vi "Intellirupter_tester.vi"() -> ()   [LabVIEW 2016]
uses:
  <vilib>/rvi/interface/nirviCloseFPGA/nirviCloseFPGA.xnode
  <vilib>/rvi/interface/nirviOpenFPGA/nirviOpenFPGA.xnode
  <vilib>/rvi/interface/nirviReadWriteControl/nirviReadWriteControl.xnode
  <vilib>/rvi/interface/Simulation/niFpgaSimulationCallBeginRW.vi
  <vilib>/rvi/errors/niLvFpgaAdjustHostInterfaceError.vi
  FPGA Bitfiles/IntelliRupter_calibrated.lvbitx
  NiFpgaLv.dll
  <vilib>/Utility/error.llb/Error Cluster From Error Code.vi
  <vilib>/FPGAPlugInAG/Dynamic/niLvFpga_Close_Dynamic.vi
  <vilib>/addons/Electrical Power/Protection/Definite Time Delay/subVIs/fpga_Time Delay Cfg.ctl
  <vilib>/addons/Electrical Power/Protection/NI_EP_Protection_FPGA.lvlib
  <vilib>/FPGAPlugInAG/cRIO-9039 (Sync)/niLvFpga_Open_cRIO-9039 (Sync).vi
  <vilib>/rvi/interface/common/dynamic/niFpgaDynamicAddResources.vi
panel:
  out "Protection settings for PV/BESS":T2
  out "dt":sgl
  out "x-y":u32
  in  "Recloser Settings":T3={"Magnitude Minimum"=0.1, "Magnitude difference level"=0.005, "Frequency difference level"=0.1, "Phase difference level"=4.0}
  out "Trip Relay8":bool=TRUE
  out "Trip Relay7":bool=TRUE
  out "Trip Relay6":bool=TRUE
  out "Trip Relay5":bool=TRUE
  out "Trip Relay4":bool=TRUE
  out "Trip Relay3":bool=TRUE
  out "Trip Relay2":bool=TRUE
  out "Trip Relay1":bool=TRUE
  out "MGCC_to_relay":bool[](array[boolean])
  out "Waveform Chart":dbl(graph)=-34.401058197021484
  in  "Count(ticks)":u32=10000
  in  "RMS minimum\nvalues":T4={"VRMS values"=[0.5, 0.5, 0.5], "IRMS values"=[0.1, 0.1, 0.1]}
  out "error out":errorcluster
  out "Relay_toMGCC":bool[](array[boolean])
  in  "Manual trip Relay8":bool
  in  "Reclose Relay8?":bool
  out "R8 Data for\ncommunication":dbl[](array[numeric])=[0.0, 0.0009045934917091171, 0.0009314979378781807, 60.0, 60.0, 28.24567985534668, 1.973525131133958e-08, -4.067070097016323e-08, 0.0, 0.0]
  in  "Manual trip Relay7":bool
  in  "Reclose Relay7?":bool
  out "R7 Data for\ncommunication":dbl[](array[numeric])=[0.0, 0.0007946116254270471, 0.0007993335901335273, 60.0, 60.0, -34.401058197021484, 1.651500881803561e-08, 8.800402599184338e-08, 0.0, 0.0]
  in  "Manual trip Relay6":bool
  in  "Reclose Relay6?":bool
  out "R6 Data for\ncommunication":dbl[](array[numeric])=[0.0, 0.0005957332732847613, 0.0007855918529021252, 60.0, 60.0, 18.105693817138672, 2.5628369915356105e-08, 3.530453627182609e-09, 0.0, 0.0]
  in  "Manual trip Relay5":bool
  in  "Reclose Relay5?":bool
  out "R5 Data for\ncommunication":dbl[](array[numeric])=[0.0, 0.0006951849487988348, 0.0008903021851711478, 60.0, 60.0, -1.4310243129730225, -8.356675233942401e-10, -1.8337251119669163e-09, 0.0, 0.0]
  in  "Manual trip Relay4":bool
  in  "Reclose Relay4?":bool
  out "R4 Data for\ncommunication":dbl[](array[numeric])=[0.0, 0.0007291746865854036, 0.0006235449784023129, 60.0, 60.0, -0.058011382818222046, -5.813950986281207e-08, -7.696689957041477e-08, 0.0, 0.0]
  in  "Manual trip Relay3":bool
  in  "Reclose Relay3?":bool
  out "R3 Data for\ncommunication":dbl[](array[numeric])=[0.0, 0.0007264402728679518, 0.0006124272449413167, 60.0, 60.0, 1.7191237211227417, 2.5547999625248733e-08, -4.286027792555224e-08, 0.0, 0.0]
  in  "Manual trip Relay2":bool
  in  "Reclose Relay2?":bool
  out "R2 Data for\ncommunication":dbl[](array[numeric])=[0.0, 0.0005227375364730379, 0.0005963174374576894, 60.0, 60.0, -1.561047911643982, -2.6251873275059558e-08, 8.429806929664172e-09, 0.0, 0.0]
  out "R1 Data for\ncommunication":dbl[](array[numeric])=[0.0, 0.0006394769755315334, 0.0006284021563432197, 60.0, 60.0, -13.953559875488281, -5.5463867419303074e-08, 7.039235159901093e-08, 0.0, 0.0]
  in  "Relay8":bool
  in  "Relay7":bool
  in  "Relay6":bool
  in  "Relay5":bool
  in  "Relay4":bool
  in  "Relay3":bool
  in  "Relay2":bool
  in  "Reclose Relay1?":bool
  out "half cycle (samples)":i32=96
  out "basic calc interval":u16=2074
  in  "stop":bool
  in  "Relay1":bool
  in  "Manual trip Relay1":bool
  # "status\nmag_left\nmag_right\nfreq_left\nfreq_right\nang_diff\nact_power\nrea_power\n0\n0"
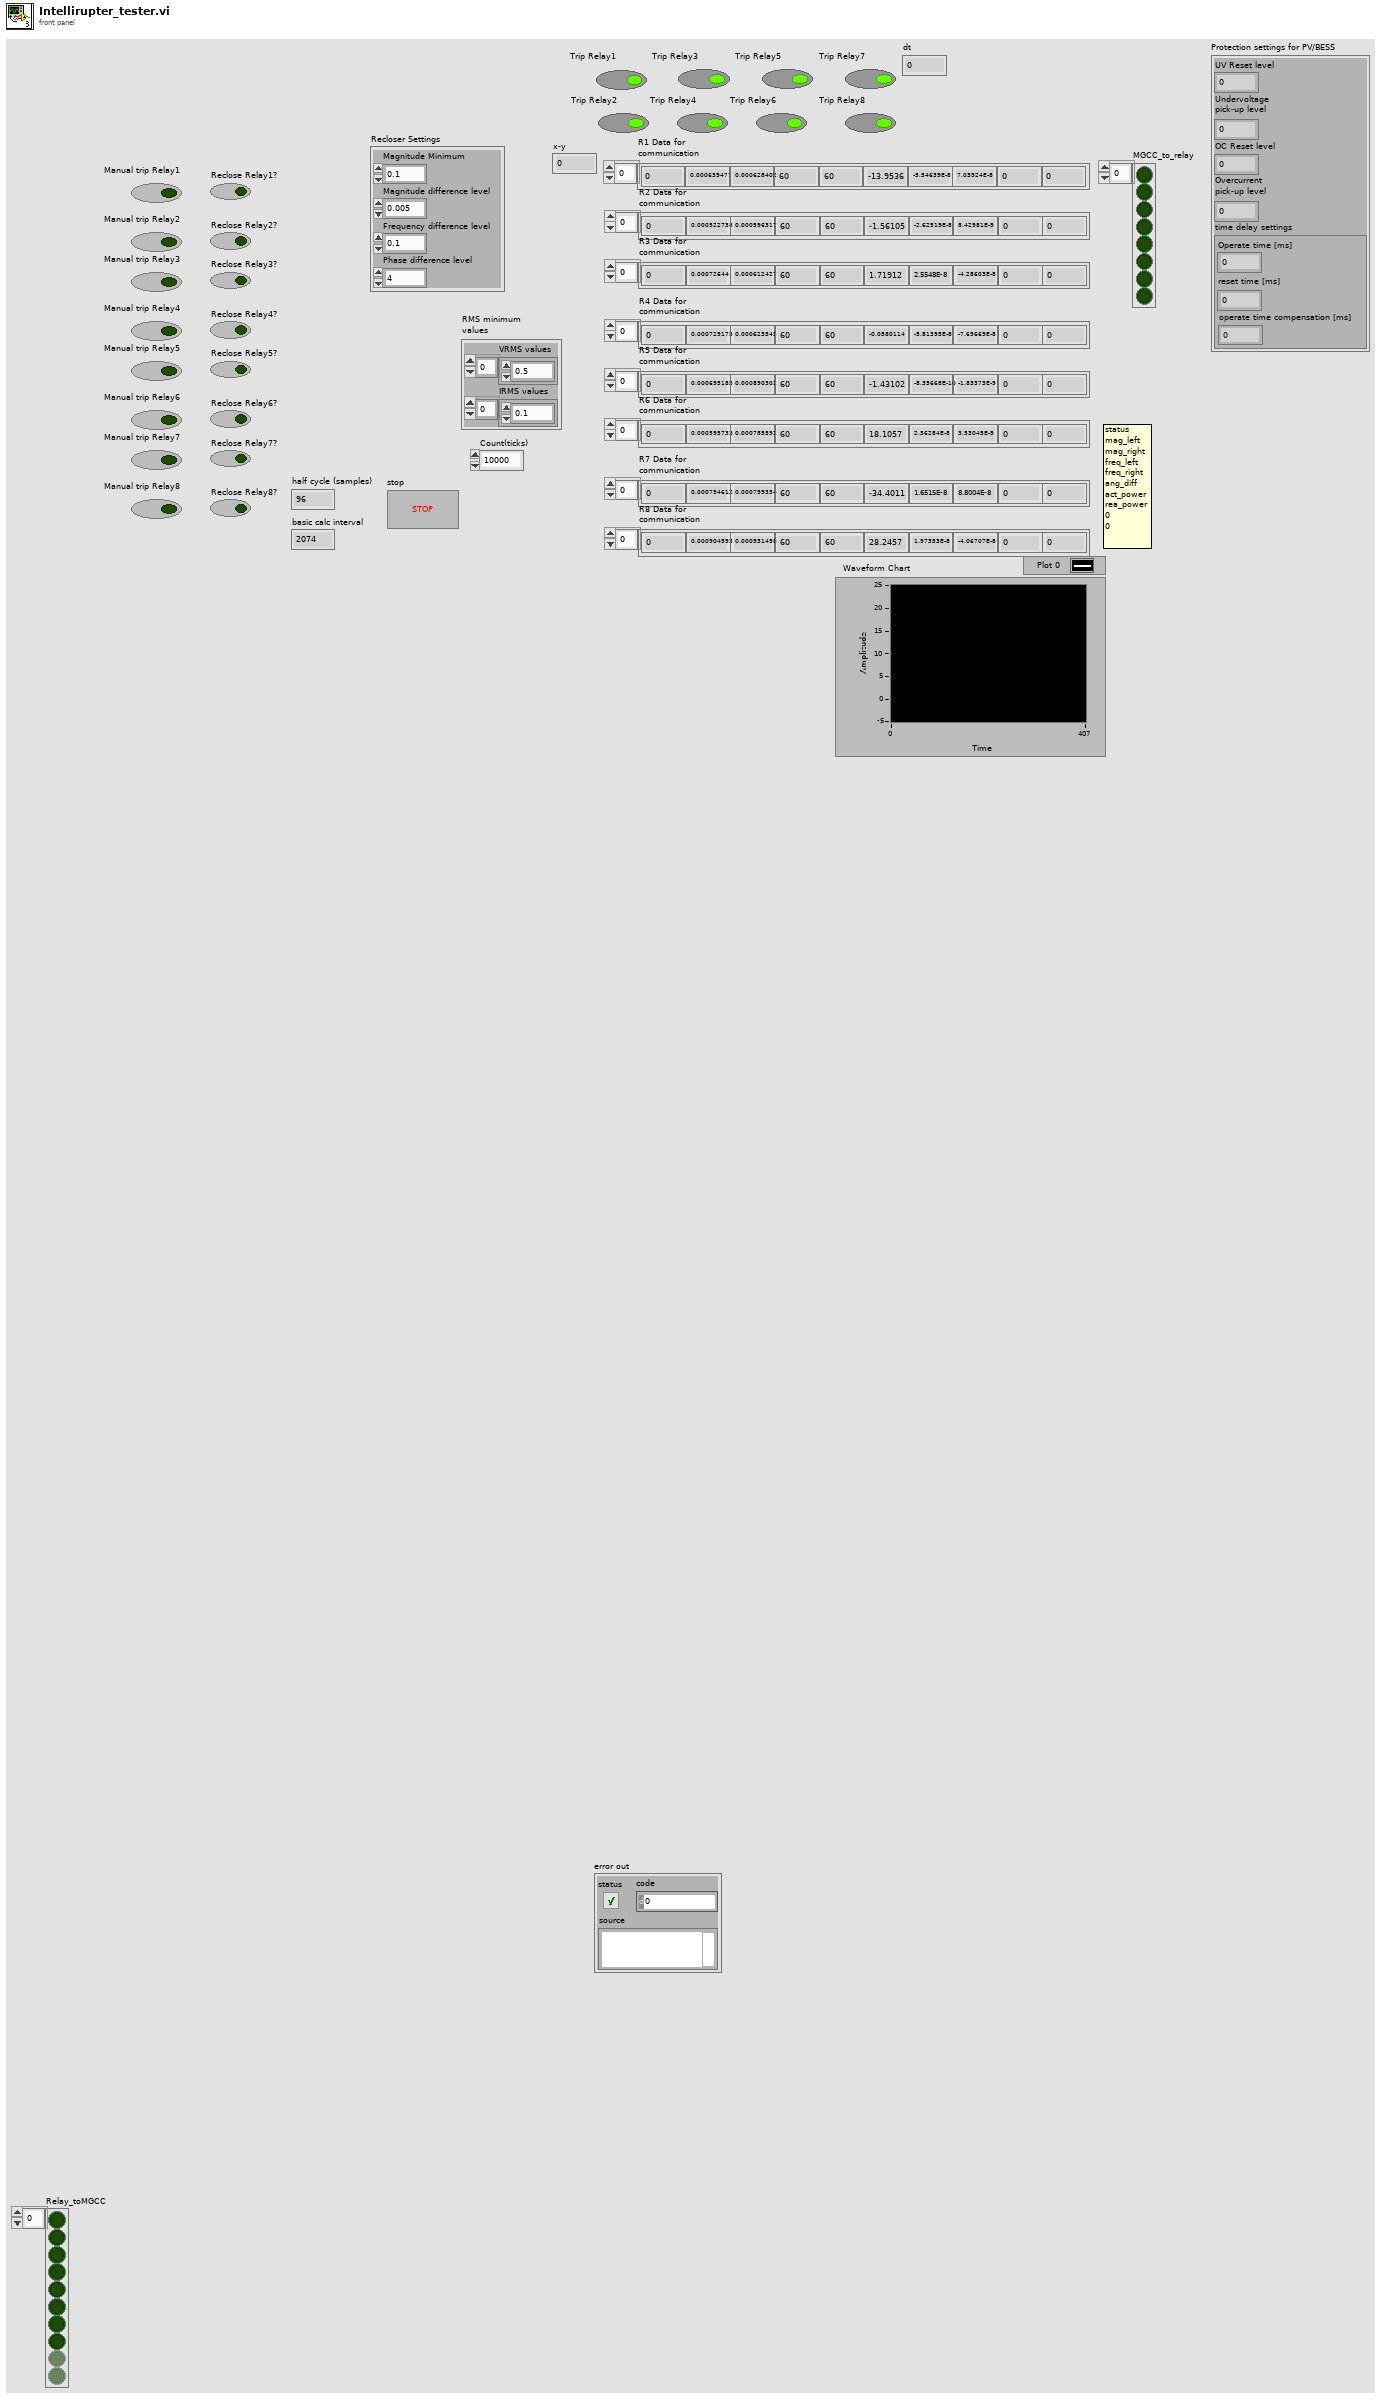
[diagram p1: front panel]
types:
  T1 = typedef "NI_EP_Protection_FPGA.lvlib/fpga_Time Delay Cfg.ctl" = cluster{"Operate time [ms]":u32, "reset time [ms]":u32, "operate time compensation [ms]":u32}
  T2 = cluster{"UV Reset level":dbl, "Undervoltage \npick-up level":dbl, "OC Reset level":dbl, "Overcurrent\npick-up level":dbl, "time delay settings":T1}
  T3 = cluster{"Magnitude Minimum":dbl, "Magnitude difference level":dbl, "Frequency difference level":dbl, "Phase difference level":dbl}
  T4 = cluster{"VRMS values":dbl[], "IRMS values":dbl[]}
  T5 = cluster{fxp<+/-,53,11>[], fxp<+/-,53,11>[], fxp<+/-,53,11>[], fxp<+/-,53,11>[], fxp<+/-,53,11>[], fxp<+/-,53,11>[], fxp<+/-,53,11>[], fxp<+/-,53,11>[], fxp<+/-,53,11>[]}
  T6 = cluster{"RMS values":dbl[], "RMS values":dbl[], "RMS values":dbl[]}
  T7 = typedef "NI_EP_Protection_FPGA.lvlib/fpga_Timer Feedback Var.ctl" = cluster{"time elapsed":u32, "start time of trip counting":u32, "start time of reseting":u32}
  T8 = typedef "NI_EP_Protection_FPGA.lvlib/fpga_State.ctl" = enum16{"Idle", "Trip Counting", "Tripped", "Reset Counting"}
  T9 = cluster{bool, bool, "Boolean":bool, "timing values out":T7, "status out":T8, "trip signal out":bool}
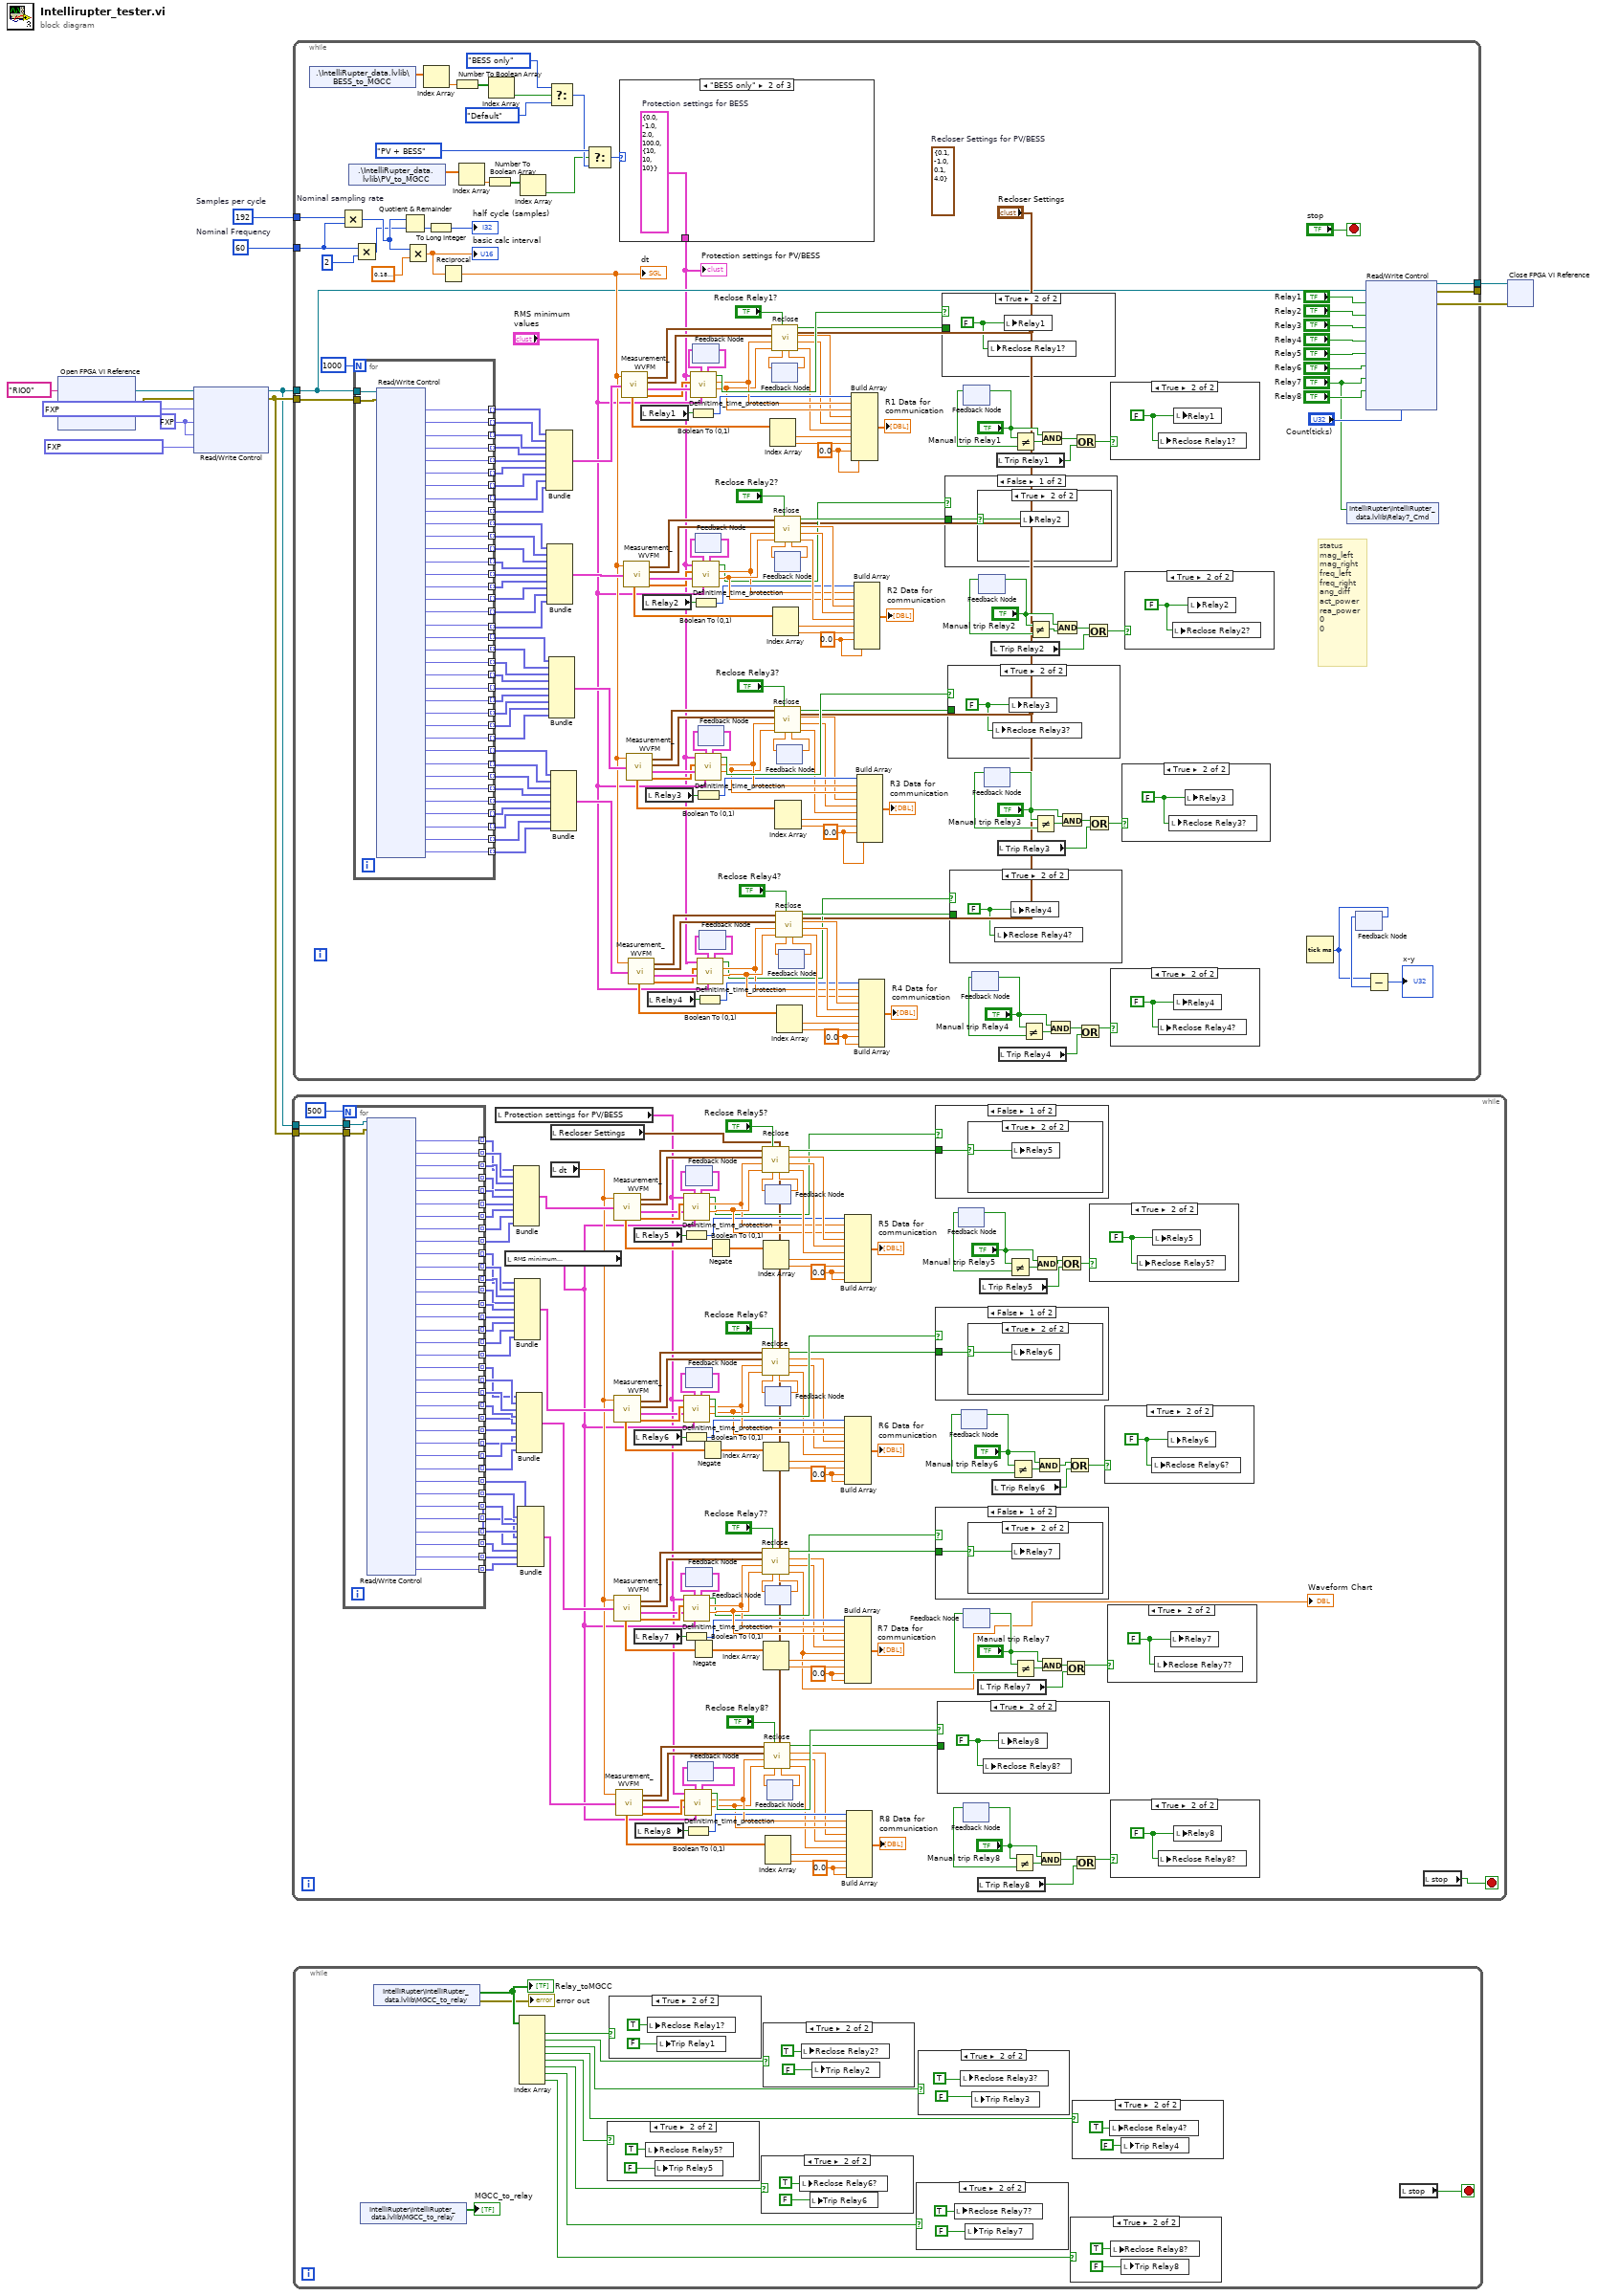
[diagram p0: block diagram]
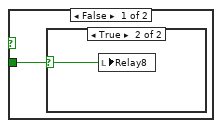
[diagram p2: hidden frame]
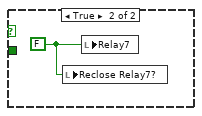
[diagram p6: hidden frame]
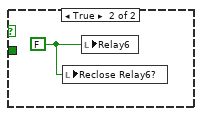
[diagram p9: hidden frame]
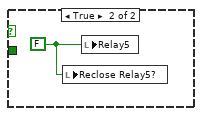
[diagram p12: hidden frame]
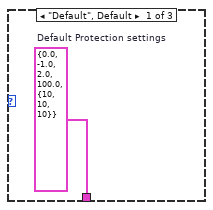
[diagram p14: hidden frame]
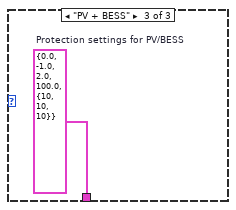
[diagram p15: hidden frame]
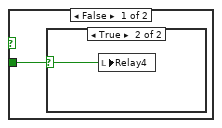
[diagram p16: hidden frame]
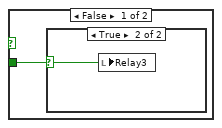
[diagram p19: hidden frame]
diagram:
  w4 = fxp<+/-,52,10> 0.0 ("I offset")
  w3 = 192  # Samples per cycle
  w10 = 60  # Nominal Frequency
  n1 = xnode "Open FPGA VI Reference"("resource name"=tag "RIO0") -> ("FPGA VI Reference Out"=w12:refnum<k20>, "error out"=w7:errorcluster)  [unwired: 1 in]
  n2 = xnode "Read/Write Control"("FPGA VI Reference In"=w12, "error in"=w7, "I scale factor"=fxp<+/-,26,5> 0.4850001335144043, "I offset"=w4, "V offset"=w4, "V scale factor"=fxp<+/-,26,5> 0.40000009536743164) -> ("FPGA VI Reference Out"=w1:refnum<k20>, "error out"=w2:errorcluster)
  n3 = while {
    tunnel: w2 -> [w16]
    tunnel: w1 -> [w14]
    stop <- w15 stop-if-true
    w99 = 0.0 ("element")
    w98 = 0.0 ("element")
    w53 = 0.0 ("element")
    w52 = 0.0 ("element")
    n4 = for {
      N: 500 -> [_]
      tunnel: w14 -> [w231]
      tunnel: w16 -> [w230]
      tunnel: [w229] -> w140 mode=indexing
      tunnel: [w228] -> w141 mode=indexing
      tunnel: [w227] -> w142 mode=indexing
      tunnel: [w226] -> w143 mode=indexing
      tunnel: [w225] -> w144 mode=indexing
      tunnel: [w224] -> w145 mode=indexing
      tunnel: [w223] -> w146 mode=indexing
      tunnel: [w222] -> w147 mode=indexing
      tunnel: [w221] -> w148 mode=indexing
      tunnel: [w220] -> w149 mode=indexing
      tunnel: [w219] -> w150 mode=indexing
      tunnel: [w218] -> w151 mode=indexing
      tunnel: [w217] -> w152 mode=indexing
      tunnel: [w216] -> w153 mode=indexing
      tunnel: [w215] -> w154 mode=indexing
      tunnel: [w214] -> w155 mode=indexing
      tunnel: [w213] -> w156 mode=indexing
      tunnel: [w212] -> w157 mode=indexing
      tunnel: [w211] -> w158 mode=indexing
      tunnel: [w210] -> w159 mode=indexing
      tunnel: [w209] -> w160 mode=indexing
      tunnel: [w208] -> w162 mode=indexing
      tunnel: [w207] -> w161 mode=indexing
      tunnel: [w206] -> w163 mode=indexing
      tunnel: [w205] -> w164 mode=indexing
      tunnel: [w204] -> w165 mode=indexing
      tunnel: [w203] -> w166 mode=indexing
      tunnel: [w202] -> w177 mode=indexing
      tunnel: [w201] -> w176 mode=indexing
      tunnel: [w200] -> w175 mode=indexing
      tunnel: [w199] -> w174 mode=indexing
      tunnel: [w198] -> w173 mode=indexing
      tunnel: [w197] -> w172 mode=indexing
      tunnel: [w196] -> w171 mode=indexing
      tunnel: [w195] -> w170 mode=indexing
      n5 = xnode "Read/Write Control"("FPGA VI Reference In"=w231, "error in"=w230) -> ("V5L BC"=w229:fxp<+/-,53,11>, "V5L CA"=w228:fxp<+/-,53,11>, "V5R AB"=w227:fxp<+/-,53,11>, "V5R BC"=w226:fxp<+/-,53,11>, "V5R CA"=w225:fxp<+/-,53,11>, "I5 A"=w224:fxp<+/-,53,11>, "I5 B"=w223:fxp<+/-,53,11>, "I5 C"=w222:fxp<+/-,53,11>, "V6L AB"=w221:fxp<+/-,53,11>, "V6L BC"=w220:fxp<+/-,53,11>, "V6L CA"=w219:fxp<+/-,53,11>, "V6R AB"=w218:fxp<+/-,53,11>, "V6R BC"=w217:fxp<+/-,53,11>, "V6R CA"=w216:fxp<+/-,53,11>, "I6 A"=w215:fxp<+/-,53,11>, "I6 B"=w214:fxp<+/-,53,11>, "I6 C"=w213:fxp<+/-,53,11>, "V7L AB"=w212:fxp<+/-,53,11>, "V7L BC"=w211:fxp<+/-,53,11>, "V7L CA"=w210:fxp<+/-,53,11>, "V7R AB"=w209:fxp<+/-,53,11>, "V7R BC"=w208:fxp<+/-,53,11>, "V7R CA"=w207:fxp<+/-,53,11>, "I7 A"=w206:fxp<+/-,53,11>, "I7 B"=w205:fxp<+/-,53,11>, "I7 C"=w204:fxp<+/-,53,11>, "V8L AB"=w203:fxp<+/-,53,11>, "V8L BC"=w202:fxp<+/-,53,11>, "V8L CA"=w201:fxp<+/-,53,11>, "V8R AB"=w200:fxp<+/-,53,11>, "V8R BC"=w199:fxp<+/-,53,11>, "V8R CA"=w198:fxp<+/-,53,11>, "I8 A"=w197:fxp<+/-,53,11>, "I8 B"=w196:fxp<+/-,53,11>, "I8 C"=w195:fxp<+/-,53,11>)  [unwired: 2 out]
    }
    n6 = local read "Protection settings for PV/BESS"() -> (w13:T2)
    n7 = local read "RMS minimum\nvalues"() -> (w17:T4)
    n8 = Bundle(w140, w141, w142, w143, w144, w145, w146, w147, w148) -> (w167:T5)  [unwired: 1 in]
    n9 = Bundle(w149, w150, w151, w152, w153, w154, w155, w156, w157) -> (w168:T5)  [unwired: 1 in]
    n10 = Bundle(w158, w159, w160, w162, w161, w163, w164, w165, w166) -> (w169:T5)  [unwired: 1 in]
    n11 = Bundle(w177, w176, w175, w175, w174, w173, w172, w171, w170) -> (w178:T5)  [unwired: 1 in]
    n12 = local read "Recloser Settings"() -> (w18:T3)
    n13 = local read "dt"() -> (w19:sgl)
    n14 = call "Measurement_WVFM.vi"("dt"=w19, "Input cluster"=w167) -> ("Total power values"=w49:dbl[], "VL array"=w33:waveform(sgl)[], "VR array"=w34:waveform(sgl)[], "RMS values"=w32:T6, "Active Power"=w133:dbl[])  [unwired: 2 in]
    n15 = call "Measurement_WVFM.vi"("dt"=w19, "Input cluster"=w168) -> ("Total power values"=w77:dbl[], "VL array"=w71:waveform(sgl)[], "VR array"=w70:waveform(sgl)[], "RMS values"=w72:T6, "Active Power"=w134:dbl[])  [unwired: 2 in]
    n16 = call "Measurement_WVFM.vi"("dt"=w19, "Input cluster"=w169) -> ("Total power values"=w78:dbl[], "VL array"=w84:waveform(sgl)[], "VR array"=w85:waveform(sgl)[], "RMS values"=w83:T6, "Active Power"=w135:dbl[])  [unwired: 2 in]
    n17 = call "Measurement_WVFM.vi"("dt"=w19, "Input cluster"=w178) -> ("Total power values"=w123:dbl[], "VL array"=w117:waveform(sgl)[], "VR array"=w116:waveform(sgl)[], "RMS values"=w118:T6, "Active Power"=w136:dbl[])  [unwired: 2 in]
    n18 = local read "Relay5"() -> (w42:bool)
    n19 = local read "Relay6"() -> (w62:bool)
    n20 = local read "Relay7"() -> (w93:bool)
    n21 = local read "Relay8"() -> (w108:bool)
    n22 = Boolean To (0,1)(Boolean=w42) -> (0, 1=w44:i16)
    n23 = Boolean To (0,1)(Boolean=w62) -> (0, 1=w60:i16)
    n24 = Boolean To (0,1)(Boolean=w93) -> (0, 1=w95:i16)
    n25 = Boolean To (0,1)(Boolean=w108) -> (0, 1=w106:i16)
    n26 = feedback #1() -> (w36:T9)  [unwired: 1 in]
    n27 = call "Definitime_time_protection.vi"("RMS minimum\nvalues"=w17, "input cluster"=w36, "RMS values"=w32, "Active Power"=w133, "Protection settings"=w13) -> ("VR RMS"=w45:dbl, "VL RMS"=w43:dbl, "trip signal"=w40:bool, "output cluster"=w35:T9)  [unwired: 1 in, 2 out]
    n28 = feedback-in #1(w35) -> ()
    n29 = feedback #2() -> (w68:T9)  [unwired: 1 in]
    n30 = call "Definitime_time_protection.vi"("RMS minimum\nvalues"=w17, "input cluster"=w68, "RMS values"=w72, "Active Power"=w134, "Protection settings"=w13) -> ("VR RMS"=w59:dbl, "VL RMS"=w61:dbl, "trip signal"=w64:bool, "output cluster"=w69:T9)  [unwired: 1 in, 2 out]
    n31 = feedback-in #2(w69) -> ()
    n32 = feedback #3() -> (w87:T9)  [unwired: 1 in]
    n33 = call "Definitime_time_protection.vi"("RMS minimum\nvalues"=w17, "input cluster"=w87, "RMS values"=w83, "Active Power"=w135, "Protection settings"=w13) -> ("VR RMS"=w96:dbl, "VL RMS"=w94:dbl, "trip signal"=w91:bool, "output cluster"=w86:T9)  [unwired: 1 in, 2 out]
    n34 = feedback-in #3(w86) -> ()
    n35 = feedback #4() -> (w114:T9)  [unwired: 1 in]
    n36 = call "Definitime_time_protection.vi"("RMS minimum\nvalues"=w17, "input cluster"=w114, "RMS values"=w118, "Active Power"=w136, "Protection settings"=w13) -> ("VR RMS"=w105:dbl, "VL RMS"=w107:dbl, "trip signal"=w110:bool, "output cluster"=w115:T9)  [unwired: 1 in, 2 out]
    n37 = feedback-in #4(w115) -> ()
    n38 = Negate(x=w78) -> (-x=w137:dbl[])
    n39 = Negate(x=w77) -> (-x=w138:dbl[])
    n40 = Negate(x=w49) -> (-x=w139:dbl[])
    n41 = Index Array(array=w139) -> (element #1=w50:dbl, element #2=w51:dbl)  [unwired: 2 in]
    n42 = Index Array(array=w138) -> (element #1=w55:dbl, element #2=w54:dbl)  [unwired: 2 in]
    n43 = Index Array(array=w137) -> (element #1=w124:dbl, element #2=w97:dbl)  [unwired: 2 in]
    n44 = feedback #5() -> (w38:dbl)  [unwired: 1 in]
    n45 = call "Reclose.vi"("Recloser Settings"=w18, "Counter In"=w38, "Reclose?"="Reclose Relay5?", "VR RMS avg"=w45, "VL RMS avg"=w43, "VR array"=w34, "VL array"=w33) -> ("Phase difference"=w48:dbl, "VR Frequency"=w47:dbl, "VL Frequency"=w46:dbl, "Recloser action"=w41:bool, "Counter Out"=w37:dbl)
    n46 = feedback-in #5(w37) -> ()
    n47 = feedback #6() -> (w66:dbl)  [unwired: 1 in]
    n48 = call "Reclose.vi"("Recloser Settings"=w18, "Counter In"=w66, "Reclose?"="Reclose Relay6?", "VR RMS avg"=w59, "VL RMS avg"=w61, "VR array"=w70, "VL array"=w71) -> ("Phase difference"=w56:dbl, "VR Frequency"=w57:dbl, "VL Frequency"=w58:dbl, "Recloser action"=w63:bool, "Counter Out"=w67:dbl)
    n49 = feedback-in #6(w67) -> ()
    n50 = feedback #7() -> (w89:dbl)  [unwired: 1 in]
    n51 = call "Reclose.vi"("Recloser Settings"=w18, "Counter In"=w89, "Reclose?"="Reclose Relay7?", "VR RMS avg"=w96, "VL RMS avg"=w94, "VR array"=w85, "VL array"=w84) -> ("Phase difference"=w24:dbl, "VR Frequency"=w26:dbl, "VL Frequency"=w25:dbl, "Recloser action"=w92:bool, "Counter Out"=w88:dbl)
    "Waveform Chart" <- w24
    n52 = feedback-in #7(w88) -> ()
    n53 = Index Array(array=w123) -> (element #1=w101:dbl, element #2=w100:dbl)  [unwired: 2 in]
    n54 = feedback #8() -> (w112:dbl)  [unwired: 1 in]
    n55 = call "Reclose.vi"("Recloser Settings"=w18, "Counter In"=w112, "Reclose?"="Reclose Relay8?", "VR RMS avg"=w105, "VL RMS avg"=w107, "VR array"=w116, "VL array"=w117) -> ("Phase difference"=w102:dbl, "VR Frequency"=w103:dbl, "VL Frequency"=w104:dbl, "Recloser action"=w109:bool, "Counter Out"=w113:dbl)
    n56 = feedback-in #8(w113) -> ()
    n57 = Build Array(w44, w43, w45, w46, w47, w48, w50, w51, w52, w52) -> (→"R5 Data for\ncommunication":dbl[])
    n58 = Build Array(w60, w61, w59, w58, w57, w56, w55, w54, w53, w53) -> (→"R6 Data for\ncommunication":dbl[])
    n59 = Build Array(w95, w94, w96, w25, w26, w24, w124, w97, w98, w98) -> (→"R7 Data for\ncommunication":dbl[])
    n60 = Build Array(w106, w107, w105, w104, w103, w102, w101, w100, w99, w99) -> (→"R8 Data for\ncommunication":dbl[])
    n61 = case shown="False" w40 {
      tunnel: w41 -> [w191 _]
      frame False {
        n62 = case shown="True" w191 {
          selector: w191 -> [_ w192]
          frame False {
          }
          frame True {
            n63 = local write "Relay5"(w192) -> ()
          }
        }
      }
      frame True {
        w193 = FALSE ("Relay7")
        n64 = local write "Reclose Relay5?"(w193) -> ()
        n65 = local write "Relay5"(w193) -> ()
      }
    }
    n66 = case shown="False" w64 {
      tunnel: w63 -> [w187 _]
      frame False {
        n67 = case shown="True" w187 {
          selector: w187 -> [_ w188]
          frame False {
          }
          frame True {
            n68 = local write "Relay6"(w188) -> ()
          }
        }
      }
      frame True {
        w189 = FALSE ("Relay7")
        n69 = local write "Reclose Relay6?"(w189) -> ()
        n70 = local write "Relay6"(w189) -> ()
      }
    }
    n71 = case shown="False" w91 {
      tunnel: w92 -> [w183 _]
      frame False {
        n72 = case shown="True" w183 {
          selector: w183 -> [_ w184]
          frame False {
          }
          frame True {
            n73 = local write "Relay7"(w184) -> ()
          }
        }
      }
      frame True {
        w185 = FALSE ("Relay7")
        n74 = local write "Reclose Relay7?"(w185) -> ()
        n75 = local write "Relay7"(w185) -> ()
      }
    }
    n76 = case shown="True" w110 {
      tunnel: w109 -> [w179 _]
      frame False {
        n77 = case shown="True" w179 {
          selector: w179 -> [_ w180]
          frame False {
          }
          frame True {
            n78 = local write "Relay8"(w180) -> ()
          }
        }
      }
      frame True {
        w181 = FALSE ("Relay7")
        n79 = local write "Reclose Relay8?"(w181) -> ()
        n80 = local write "Relay8"(w181) -> ()
      }
    }
    n81 = feedback #9() -> (w28:bool)  [unwired: 1 in]
    n82 = feedback-in #9("Manual trip Relay5") -> ()
    n83 = feedback #10() -> (w76:bool)  [unwired: 1 in]
    n84 = feedback-in #10("Manual trip Relay6") -> ()
    n85 = feedback #11() -> (w122:bool)  [unwired: 1 in]
    n86 = feedback-in #11("Manual trip Relay8") -> ()
    n87 = feedback #12() -> (w79:bool)  [unwired: 1 in]
    n88 = feedback-in #12("Manual trip Relay7") -> ()
    n89 = local read "Trip Relay8"() -> (w126:bool)
    n90 = local read "Trip Relay7"() -> (w128:bool)
    n91 = local read "Trip Relay5"() -> (w132:bool)
    n92 = local read "Trip Relay6"() -> (w130:bool)
    n93 = Not Equal?(x="Manual trip Relay5", y=w28) -> (x != y?=w29:bool)
    n94 = Not Equal?(x="Manual trip Relay6", y=w76) -> (x != y?=w75:bool)
    n95 = Not Equal?(x="Manual trip Relay8", y=w122) -> (x != y?=w121:bool)
    n96 = Not Equal?(x="Manual trip Relay7", y=w79) -> (x != y?=w80:bool)
    n97 = And(x="Manual trip Relay5", y=w29) -> (x .and. y?=w31:bool)
    n98 = And(x="Manual trip Relay6", y=w75) -> (x .and. y?=w73:bool)
    n99 = And(x="Manual trip Relay8", y=w121) -> (x .and. y?=w119:bool)
    n100 = And(x="Manual trip Relay7", y=w80) -> (x .and. y?=w82:bool)
    n101 = Or(x=w31, y=w132) -> (x .or. y?=w131:bool)
    n102 = Or(x=w82, y=w128) -> (x .or. y?=w127:bool)
    n103 = Or(x=w73, y=w130) -> (x .or. y?=w129:bool)
    n104 = Or(x=w119, y=w126) -> (x .or. y?=w125:bool)
    n105 = case shown="True" w131 {
      frame False {
      }
      frame True {
        w194 = FALSE ("Relay7")
        n106 = local write "Reclose Relay5?"(w194) -> ()
        n107 = local write "Relay5"(w194) -> ()
      }
    }
    n108 = case shown="True" w129 {
      frame False {
      }
      frame True {
        w190 = FALSE ("Relay7")
        n109 = local write "Reclose Relay6?"(w190) -> ()
        n110 = local write "Relay6"(w190) -> ()
      }
    }
    n111 = case shown="True" w127 {
      frame False {
      }
      frame True {
        w186 = FALSE ("Relay7")
        n112 = local write "Reclose Relay7?"(w186) -> ()
        n113 = local write "Relay7"(w186) -> ()
      }
    }
    n114 = case shown="True" w125 {
      frame False {
      }
      frame True {
        w182 = FALSE ("Relay7")
        n115 = local write "Reclose Relay8?"(w182) -> ()
        n116 = local write "Relay8"(w182) -> ()
      }
    }
    n117 = local read "stop"() -> (w15:bool)
  }
  n118 = while {
    tunnel: w1 -> [w234]
    tunnel: w10 -> [w424]
    tunnel: [w422] -> w9
    tunnel: [w421] -> w8
    tunnel: w2 -> [w233]
    tunnel: w3 -> [w266]
    stop <- "stop" stop-if-true
    (unwired) T3 {"Magnitude Minimum"=0.1, "Magnitude difference level"=-1.0, "Frequency difference level"=0.1, "Phase difference level"=4.0}  # Recloser Settings for PV/BESS
    w308 = 0.0 ("element")
    w318 = 0.0 ("element")
    w368 = 0.0 ("element")
    w384 = 0.0 ("element")
    # "status\nmag_left\nmag_right\nfreq_left\nfreq_right\nang_diff\nact_power\nrea_power\n0\n0"
    n119 = shared-variable ".\\IntelliRupter_data.lvlib\\BESS_to_MGCC"() -> (w240:dbl[])  [unwired: 1 in, 1 out]
    n120 = Multiply "Nominal sampling rate"(x=w266, y=w424) -> (x*y=w430:i32)
    n121 = shared-variable ".\\IntelliRupter_data.lvlib\\PV_to_MGCC"() -> (w244:dbl[])  [unwired: 1 in, 1 out]
    n122 = Multiply(x=w424, y=2) -> (x*y=w426:i32)
    n123 = for {
      N: 1000 -> [_]
      tunnel: w234 -> [w484]
      tunnel: w233 -> [w483]
      tunnel: [w482] -> w415 mode=indexing
      tunnel: [w481] -> w414 mode=indexing
      tunnel: [w480] -> w413 mode=indexing
      tunnel: [w479] -> w412 mode=indexing
      tunnel: [w478] -> w411 mode=indexing
      tunnel: [w477] -> w410 mode=indexing
      tunnel: [w476] -> w409 mode=indexing
      tunnel: [w475] -> w408 mode=indexing
      tunnel: [w474] -> w407 mode=indexing
      tunnel: [w473] -> w377 mode=indexing
      tunnel: [w472] -> w376 mode=indexing
      tunnel: [w471] -> w375 mode=indexing
      tunnel: [w470] -> w374 mode=indexing
      tunnel: [w469] -> w373 mode=indexing
      tunnel: [w468] -> w372 mode=indexing
      tunnel: [w467] -> w371 mode=indexing
      tunnel: [w466] -> w370 mode=indexing
      tunnel: [w465] -> w369 mode=indexing
      tunnel: [w464] -> w317 mode=indexing
      tunnel: [w463] -> w316 mode=indexing
      tunnel: [w462] -> w315 mode=indexing
      tunnel: [w461] -> w314 mode=indexing
      tunnel: [w460] -> w313 mode=indexing
      tunnel: [w459] -> w312 mode=indexing
      tunnel: [w458] -> w311 mode=indexing
      tunnel: [w457] -> w310 mode=indexing
      tunnel: [w456] -> w309 mode=indexing
      tunnel: [w455] -> w282 mode=indexing
      tunnel: [w454] -> w281 mode=indexing
      tunnel: [w453] -> w280 mode=indexing
      tunnel: [w452] -> w279 mode=indexing
      tunnel: [w451] -> w278 mode=indexing
      tunnel: [w450] -> w277 mode=indexing
      tunnel: [w449] -> w276 mode=indexing
      tunnel: [w448] -> w275 mode=indexing
      tunnel: [w447] -> w274 mode=indexing
      n124 = xnode "Read/Write Control"("FPGA VI Reference In"=w484, "error in"=w483) -> ("V1L AB"=w482:fxp<+/-,53,11>, "V1L BC"=w481:fxp<+/-,53,11>, "V1L CA"=w480:fxp<+/-,53,11>, "V1R AB"=w479:fxp<+/-,53,11>, "V1R BC"=w478:fxp<+/-,53,11>, "V1R CA"=w477:fxp<+/-,53,11>, "I1 A"=w476:fxp<+/-,53,11>, "I1 B"=w475:fxp<+/-,53,11>, "I1 C"=w474:fxp<+/-,53,11>, "V2L AB"=w473:fxp<+/-,53,11>, "V2L BC"=w472:fxp<+/-,53,11>, "V2L CA"=w471:fxp<+/-,53,11>, "V2R AB"=w470:fxp<+/-,53,11>, "V2R BC"=w469:fxp<+/-,53,11>, "V2R CA"=w468:fxp<+/-,53,11>, "I2 A"=w467:fxp<+/-,53,11>, "I2 B"=w466:fxp<+/-,53,11>, "I2 C"=w465:fxp<+/-,53,11>, "V3L AB"=w464:fxp<+/-,53,11>, "V3L BC"=w463:fxp<+/-,53,11>, "V3L CA"=w462:fxp<+/-,53,11>, "V3R AB"=w461:fxp<+/-,53,11>, "V3R BC"=w460:fxp<+/-,53,11>, "V3R CA"=w459:fxp<+/-,53,11>, "I3 A"=w458:fxp<+/-,53,11>, "I3 B"=w457:fxp<+/-,53,11>, "I3 C"=w456:fxp<+/-,53,11>, "V4L AB"=w455:fxp<+/-,53,11>, "V4L BC"=w454:fxp<+/-,53,11>, "V4L CA"=w453:fxp<+/-,53,11>, "V4R AB"=w452:fxp<+/-,53,11>, "V4R BC"=w451:fxp<+/-,53,11>, "V4R CA"=w450:fxp<+/-,53,11>, "I4 A"=w449:fxp<+/-,53,11>, "I4 B"=w448:fxp<+/-,53,11>, "I4 C"=w447:fxp<+/-,53,11>)  [unwired: 2 out]
    }
    n125 = Quotient & Remainder(x=w430, y=w426) -> (floor(x/y)=w428:i32)  [unwired: 1 out]
    n126 = Multiply(x=w430, y=sgl 0.18) -> (x*y=w431:sgl)
    "basic calc interval" <- w431
    n127 = Index Array(array=w240) -> (element=w239:dbl)  [unwired: 1 in]
    n128 = To Long Integer(number=w428) -> (32bit integer=→"half cycle (samples)":i32)
    n129 = Reciprocal(x=w431) -> (1/x=w273:sgl)
    "dt" <- w273
    n130 = Number To Boolean Array(number=w239) -> (Boolean array=w248:bool[])
    n131 = Index Array(array=w244) -> (element=w243:dbl)  [unwired: 1 in]
    n132 = Number To Boolean Array(number=w243) -> (Boolean array=w242:bool[])
    n133 = Index Array(array=w248) -> (element=w247:bool)  [unwired: 1 in]
    n134 = Index Array(array=w242) -> (element=w241:bool)  [unwired: 1 in]
    n135 = Bundle(w415, w414, w413, w412, w411, w410, w409, w408, w407) -> (w406:T5)  [unwired: 1 in]
    n136 = Bundle(w377, w376, w375, w374, w373, w372, w371, w370, w369) -> (w343:T5)  [unwired: 1 in]
    n137 = Select(t=enum16{"Default", "BESS only", "PV + BESS"}."BESS only", s=w247, f=enum16{"Default", "BESS only", "PV + BESS"}."Default") -> (s? t:f=w249:enum16{"Default", "BESS only", "PV + BESS"})
    n138 = Bundle(w317, w316, w315, w314, w313, w312, w311, w310, w309) -> (w342:T5)  [unwired: 1 in]
    n139 = Bundle(w282, w281, w280, w279, w278, w277, w276, w275, w274) -> (w283:T5)  [unwired: 1 in]
    n140 = Select(t=enum16{"Default", "BESS only", "PV + BESS"}."PV + BESS", s=w241, f=w249) -> (s? t:f=w251:enum16{"Default", "BESS only", "PV + BESS"})
    n141 = case shown="\"BESS only\"" w251 {
      tunnel: [w432 w433 w434] -> w232
      frame "Default", Default {
        w432 = T2 {"UV Reset level"=0.0, "Undervoltage \npick-up level"=-1.0, "OC Reset level"=2.0, "Overcurrent\npick-up level"=100.0, "time delay settings"={"Operate time [ms]"=10, "reset time [ms]"=10, "operate time compensation [ms]"=10}}  # Default Protection settings
      }
      frame "BESS only" {
        w433 = T2 {"UV Reset level"=0.0, "Undervoltage \npick-up level"=-1.0, "OC Reset level"=2.0, "Overcurrent\npick-up level"=100.0, "time delay settings"={"Operate time [ms]"=10, "reset time [ms]"=10, "operate time compensation [ms]"=10}}  # Protection settings for BESS
      }
      frame "PV + BESS" {
        w434 = T2 {"UV Reset level"=0.0, "Undervoltage \npick-up level"=-1.0, "OC Reset level"=2.0, "Overcurrent\npick-up level"=100.0, "time delay settings"={"Operate time [ms]"=10, "reset time [ms]"=10, "operate time compensation [ms]"=10}}  # Protection settings for PV/BESS
      }
    }
    "Protection settings for PV/BESS" <- w232
    n142 = call "Measurement_WVFM.vi"("dt"=w273, "Input cluster"=w406) -> ("Total power values"=w387:dbl[], "VL array"=w404:waveform(sgl)[], "VR array"=w403:waveform(sgl)[], "RMS values"=w405:T6, "Active Power"=w256:dbl[])  [unwired: 2 in]
    n143 = call "Measurement_WVFM.vi"("dt"=w273, "Input cluster"=w343) -> ("Total power values"=w365:dbl[], "VL array"=w349:waveform(sgl)[], "VR array"=w350:waveform(sgl)[], "RMS values"=w348:T6, "Active Power"=w255:dbl[])  [unwired: 2 in]
    n144 = call "Measurement_WVFM.vi"("dt"=w273, "Input cluster"=w342) -> ("Total power values"=w320:dbl[], "VL array"=w336:waveform(sgl)[], "VR array"=w335:waveform(sgl)[], "RMS values"=w337:T6, "Active Power"=w254:dbl[])  [unwired: 2 in]
    n145 = call "Measurement_WVFM.vi"("dt"=w273, "Input cluster"=w283) -> ("Total power values"=w305:dbl[], "VL array"=w289:waveform(sgl)[], "VR array"=w290:waveform(sgl)[], "RMS values"=w288:T6, "Active Power"=w253:dbl[])  [unwired: 2 in]
    n146 = local read "Relay1"() -> (w394:bool)
    n147 = local read "Relay2"() -> (w358:bool)
    n148 = local read "Relay3"() -> (w327:bool)
    n149 = local read "Relay4"() -> (w298:bool)
    n150 = Boolean To (0,1)(Boolean=w394) -> (0, 1=w392:i16)
    n151 = feedback #13() -> (w401:T9)  [unwired: 1 in]
    n152 = call "Definitime_time_protection.vi"("RMS minimum\nvalues"="RMS minimum\nvalues", "input cluster"=w401, "RMS values"=w405, "Active Power"=w256, "Protection settings"=w232) -> ("VR RMS"=w391:dbl, "VL RMS"=w393:dbl, "trip signal"=w397:bool, "output cluster"=w402:T9)  [unwired: 1 in, 2 out]
    n153 = feedback-in #13(w402) -> ()
    n154 = Boolean To (0,1)(Boolean=w358) -> (0, 1=w360:i16)
    n155 = feedback #14() -> (w352:T9)  [unwired: 1 in]
    n156 = call "Definitime_time_protection.vi"("RMS minimum\nvalues"="RMS minimum\nvalues", "input cluster"=w352, "RMS values"=w348, "Active Power"=w255, "Protection settings"=w232) -> ("VR RMS"=w361:dbl, "VL RMS"=w359:dbl, "trip signal"=w356:bool, "output cluster"=w351:T9)  [unwired: 1 in, 2 out]
    n157 = feedback-in #14(w351) -> ()
    n158 = Boolean To (0,1)(Boolean=w327) -> (0, 1=w325:i16)
    n159 = Boolean To (0,1)(Boolean=w298) -> (0, 1=w300:i16)
    n160 = feedback #15() -> (w333:T9)  [unwired: 1 in]
    n161 = call "Definitime_time_protection.vi"("RMS minimum\nvalues"="RMS minimum\nvalues", "input cluster"=w333, "RMS values"=w337, "Active Power"=w254, "Protection settings"=w232) -> ("VR RMS"=w324:dbl, "VL RMS"=w326:dbl, "trip signal"=w329:bool, "output cluster"=w334:T9)  [unwired: 1 in, 2 out]
    n162 = feedback-in #15(w334) -> ()
    n163 = feedback #16() -> (w292:T9)  [unwired: 1 in]
    n164 = call "Definitime_time_protection.vi"("RMS minimum\nvalues"="RMS minimum\nvalues", "input cluster"=w292, "RMS values"=w288, "Active Power"=w253, "Protection settings"=w232) -> ("VR RMS"=w301:dbl, "VL RMS"=w299:dbl, "trip signal"=w296:bool, "output cluster"=w291:T9)  [unwired: 1 in, 2 out]
    n165 = feedback-in #16(w291) -> ()
    n166 = Index Array(array=w387) -> (element #1=w386:dbl, element #2=w385:dbl)  [unwired: 2 in]
    n167 = feedback #17() -> (w399:dbl)  [unwired: 1 in]
    n168 = call "Reclose.vi"("Recloser Settings"="Recloser Settings", "Counter In"=w399, "Reclose?"="Reclose Relay1?", "VR RMS avg"=w391, "VL RMS avg"=w393, "VR array"=w403, "VL array"=w404) -> ("Phase difference"=w388:dbl, "VR Frequency"=w389:dbl, "VL Frequency"=w390:dbl, "Recloser action"=w396:bool, "Counter Out"=w400:dbl)
    n169 = feedback-in #17(w400) -> ()
    n170 = Index Array(array=w365) -> (element #1=w366:dbl, element #2=w367:dbl)  [unwired: 2 in]
    n171 = feedback #18() -> (w354:dbl)  [unwired: 1 in]
    n172 = call "Reclose.vi"("Recloser Settings"="Recloser Settings", "Counter In"=w354, "Reclose?"="Reclose Relay2?", "VR RMS avg"=w361, "VL RMS avg"=w359, "VR array"=w350, "VL array"=w349) -> ("Phase difference"=w364:dbl, "VR Frequency"=w363:dbl, "VL Frequency"=w362:dbl, "Recloser action"=w357:bool, "Counter Out"=w353:dbl)
    n173 = feedback-in #18(w353) -> ()
    n174 = Index Array(array=w320) -> (element #1=w265:dbl, element #2=w319:dbl)  [unwired: 2 in]
    n175 = feedback #19() -> (w331:dbl)  [unwired: 1 in]
    n176 = call "Reclose.vi"("Recloser Settings"="Recloser Settings", "Counter In"=w331, "Reclose?"="Reclose Relay3?", "VR RMS avg"=w324, "VL RMS avg"=w326, "VR array"=w335, "VL array"=w336) -> ("Phase difference"=w321:dbl, "VR Frequency"=w322:dbl, "VL Frequency"=w323:dbl, "Recloser action"=w328:bool, "Counter Out"=w332:dbl)
    n177 = feedback-in #19(w332) -> ()
    n178 = Index Array(array=w305) -> (element #1=w306:dbl, element #2=w307:dbl)  [unwired: 2 in]
    n179 = feedback #20() -> (w294:dbl)  [unwired: 1 in]
    n180 = call "Reclose.vi"("Recloser Settings"="Recloser Settings", "Counter In"=w294, "Reclose?"="Reclose Relay4?", "VR RMS avg"=w301, "VL RMS avg"=w299, "VR array"=w290, "VL array"=w289) -> ("Phase difference"=w304:dbl, "VR Frequency"=w303:dbl, "VL Frequency"=w302:dbl, "Recloser action"=w297:bool, "Counter Out"=w293:dbl)
    n181 = feedback-in #20(w293) -> ()
    n182 = Build Array(w392, w393, w391, w390, w389, w388, w386, w385, w384, w384) -> (→"R1 Data for\ncommunication":dbl[])
    n183 = Build Array(w360, w359, w361, w362, w363, w364, w366, w367, w368, w368) -> (→"R2 Data for\ncommunication":dbl[])
    n184 = Build Array(w325, w326, w324, w323, w322, w321, w265, w319, w318, w318) -> (→"R3 Data for\ncommunication":dbl[])
    n185 = Build Array(w300, w299, w301, w302, w303, w304, w306, w307, w308, w308) -> (→"R4 Data for\ncommunication":dbl[])
    n186 = case shown="True" w397 {
      tunnel: w396 -> [w485 _]
      frame False {
        n187 = case shown="True" w485 {
          selector: w485 -> [_ w486]
          frame False {
          }
          frame True {
            n188 = local write "Relay1"(w486) -> ()
          }
        }
      }
      frame True {
        w487 = FALSE ("Relay7")
        n189 = local write "Reclose Relay1?"(w487) -> ()
        n190 = local write "Relay1"(w487) -> ()
      }
    }
    n191 = case shown="False" w356 {
      tunnel: w357 -> [w443 _]
      frame False {
        n192 = case shown="True" w443 {
          selector: w443 -> [_ w444]
          frame False {
          }
          frame True {
            n193 = local write "Relay2"(w444) -> ()
          }
        }
      }
      frame True {
        w445 = FALSE ("Relay7")
        n194 = local write "Reclose Relay2?"(w445) -> ()
        n195 = local write "Relay2"(w445) -> ()
      }
    }
    n196 = case shown="True" w329 {
      tunnel: w328 -> [w439 _]
      frame False {
        n197 = case shown="True" w439 {
          selector: w439 -> [_ w440]
          frame False {
          }
          frame True {
            n198 = local write "Relay3"(w440) -> ()
          }
        }
      }
      frame True {
        w441 = FALSE ("Relay7")
        n199 = local write "Reclose Relay3?"(w441) -> ()
        n200 = local write "Relay3"(w441) -> ()
      }
    }
    n201 = case shown="True" w296 {
      tunnel: w297 -> [w435 _]
      frame False {
        n202 = case shown="True" w435 {
          selector: w435 -> [_ w436]
          frame False {
          }
          frame True {
            n203 = local write "Relay4"(w436) -> ()
          }
        }
      }
      frame True {
        w437 = FALSE ("Relay7")
        n204 = local write "Reclose Relay4?"(w437) -> ()
        n205 = local write "Relay4"(w437) -> ()
      }
    }
    n206 = feedback #21() -> (w420:bool)  [unwired: 1 in]
    n207 = feedback-in #21("Manual trip Relay1") -> ()
    n208 = feedback #22() -> (w284:bool)  [unwired: 1 in]
    n209 = feedback-in #22("Manual trip Relay4") -> ()
    n210 = feedback #23() -> (w344:bool)  [unwired: 1 in]
    n211 = feedback-in #23("Manual trip Relay2") -> ()
    n212 = feedback #24() -> (w341:bool)  [unwired: 1 in]
    n213 = feedback-in #24("Manual trip Relay3") -> ()
    n214 = local read "Trip Relay2"() -> (w259:bool)
    n215 = local read "Trip Relay1"() -> (w257:bool)
    n216 = local read "Trip Relay3"() -> (w261:bool)
    n217 = local read "Trip Relay4"() -> (w263:bool)
    n218 = Not Equal?(x="Manual trip Relay1", y=w420) -> (x != y?=w419:bool)
    n219 = Not Equal?(x="Manual trip Relay4", y=w284) -> (x != y?=w285:bool)
    n220 = Not Equal?(x="Manual trip Relay2", y=w344) -> (x != y?=w345:bool)
    n221 = Not Equal?(x="Manual trip Relay3", y=w341) -> (x != y?=w340:bool)
    n222 = And(x="Manual trip Relay1", y=w419) -> (x .and. y?=w417:bool)
    n223 = And(x="Manual trip Relay4", y=w285) -> (x .and. y?=w287:bool)
    n224 = And(x="Manual trip Relay2", y=w345) -> (x .and. y?=w347:bool)
    n225 = And(x="Manual trip Relay3", y=w340) -> (x .and. y?=w338:bool)
    n226 = Or(x=w417, y=w257) -> (x .or. y?=w258:bool)
    n227 = Or(x=w287, y=w263) -> (x .or. y?=w264:bool)
    n228 = Or(x=w347, y=w259) -> (x .or. y?=w260:bool)
    n229 = Or(x=w338, y=w261) -> (x .or. y?=w262:bool)
    n230 = case shown="True" w258 {
      frame False {
      }
      frame True {
        w488 = FALSE ("Relay7")
        n231 = local write "Reclose Relay1?"(w488) -> ()
        n232 = local write "Relay1"(w488) -> ()
      }
    }
    n233 = case shown="True" w264 {
      frame False {
      }
      frame True {
        w438 = FALSE ("Relay7")
        n234 = local write "Reclose Relay4?"(w438) -> ()
        n235 = local write "Relay4"(w438) -> ()
      }
    }
    n236 = case shown="True" w262 {
      frame False {
      }
      frame True {
        w442 = FALSE ("Relay7")
        n237 = local write "Reclose Relay3?"(w442) -> ()
        n238 = local write "Relay3"(w442) -> ()
      }
    }
    n239 = case shown="True" w260 {
      frame False {
      }
      frame True {
        w446 = FALSE ("Relay7")
        n240 = local write "Reclose Relay2?"(w446) -> ()
        n241 = local write "Relay2"(w446) -> ()
      }
    }
    n242 = Tick Count (ms)() -> (millisecond timer value=w236:u32)
    n243 = shared-variable "IntelliRupter\\IntelliRupter_data.lvlib\\Relay7_Cmd"("Relay7") -> ()  [unwired: 1 in, 1 out]
    n244 = feedback #25() -> (w237:u32)  [unwired: 1 in]
    n245 = feedback-in #25(w236) -> ()
    n246 = xnode "Read/Write Control"("FPGA VI Reference In"=w234, "Relay1"="Relay1", "Relay2"="Relay2", "Relay3"="Relay3", "Relay4"="Relay4", "Relay5"="Relay5", "Relay6"="Relay6", "Relay7"="Relay7", "Relay8"="Relay8", "Count(ticks)"="Count(ticks)") -> ("FPGA VI Reference Out"=w422:refnum<k20>, "error out"=w421:errorcluster)  [unwired: 1 in]
    n247 = Subtract(x=w236, y=w237) -> (x-y=→"x-y":u32)
  }
  n248 = while {
    stop <- w500 stop-if-true
    n249 = shared-variable "IntelliRupter\\IntelliRupter_data.lvlib\\MGCC_to_relay"() -> (→"MGCC_to_relay":bool[])  [unwired: 1 in, 1 out]
    n250 = shared-variable "IntelliRupter\\IntelliRupter_data.lvlib\\MGCC_to_relay"() -> (w491:bool[], error out=→"error out":errorcluster)  [unwired: 1 in]
    "Relay_toMGCC" <- w491
    n251 = Index Array(array=w491) -> (element #1=w492:bool, element #2=w493:bool, element #3=w494:bool, element #4=w495:bool, element #5=w496:bool, element #6=w497:bool, element #7=w498:bool, element #8=w499:bool)  [unwired: 8 in]
    n252 = case shown="True" w496 {
      frame False {
        "Trip Relay5" <- TRUE ("Manual trip Relay1")
      }
      frame True {
        n253 = local write "Reclose Relay5?"(TRUE ("Reclose Relay1?")) -> ()
        n254 = local write "Trip Relay5"(FALSE ("Reclose Relay1?")) -> ()
      }
    }
    n255 = case shown="True" w492 {
      frame False {
        "Trip Relay1" <- TRUE ("Manual trip Relay1")
      }
      frame True {
        n256 = local write "Reclose Relay1?"(TRUE ("Reclose Relay1?")) -> ()
        n257 = local write "Trip Relay1"(FALSE ("Reclose Relay1?")) -> ()
      }
    }
    n258 = case shown="True" w497 {
      frame False {
        "Trip Relay6" <- TRUE ("Manual trip Relay1")
      }
      frame True {
        n259 = local write "Reclose Relay6?"(TRUE ("Reclose Relay1?")) -> ()
        n260 = local write "Trip Relay6"(FALSE ("Reclose Relay1?")) -> ()
      }
    }
    n261 = case shown="True" w493 {
      frame False {
        "Trip Relay2" <- TRUE ("Manual trip Relay1")
      }
      frame True {
        n262 = local write "Reclose Relay2?"(TRUE ("Reclose Relay1?")) -> ()
        n263 = local write "Trip Relay2"(FALSE ("Reclose Relay1?")) -> ()
      }
    }
    n264 = case shown="True" w498 {
      frame False {
        "Trip Relay7" <- TRUE ("Manual trip Relay1")
      }
      frame True {
        n265 = local write "Reclose Relay7?"(TRUE ("Reclose Relay1?")) -> ()
        n266 = local write "Trip Relay7"(FALSE ("Reclose Relay1?")) -> ()
      }
    }
    n267 = case shown="True" w494 {
      frame False {
        "Trip Relay3" <- TRUE ("Reclose Relay1?")
      }
      frame True {
        n268 = local write "Reclose Relay3?"(TRUE ("Manual trip Relay1")) -> ()
        n269 = local write "Trip Relay3"(FALSE ("Manual trip Relay1")) -> ()
      }
    }
    n270 = case shown="True" w499 {
      frame False {
        "Trip Relay8" <- TRUE ("Manual trip Relay1")
      }
      frame True {
        n271 = local write "Reclose Relay8?"(TRUE ("Reclose Relay1?")) -> ()
        n272 = local write "Trip Relay8"(FALSE ("Reclose Relay1?")) -> ()
      }
    }
    n273 = case shown="True" w495 {
      frame False {
        "Trip Relay4" <- TRUE ("Manual trip Relay1")
      }
      frame True {
        n274 = local write "Reclose Relay4?"(TRUE ("Reclose Relay1?")) -> ()
        n275 = local write "Trip Relay4"(FALSE ("Trip Relay4")) -> ()
      }
    }
    n276 = local read "stop"() -> (w500:bool)
  }
  n277 = xnode "Close FPGA VI Reference"("FPGA VI Reference In"=w9, "error in"=w8) -> ()  [unwired: 1 out]
